vi "Sub_Seach_Changing_Point.vi"(7 "String?(F)":bool, 8 "Data Interval Time(ms)":dbl, 9 "Reverse Search?":bool, 10 "Input":string, 11 "Input Array":u32[](array[numeric])) -> (3 "Output":i32[](array[numeric]))   [LabVIEW 2015]
panel:
  out "x-y":i32[](array[numeric])
  out "Waveform Graph":u32[][](graph)
  out "Array":i32[](array[numeric])
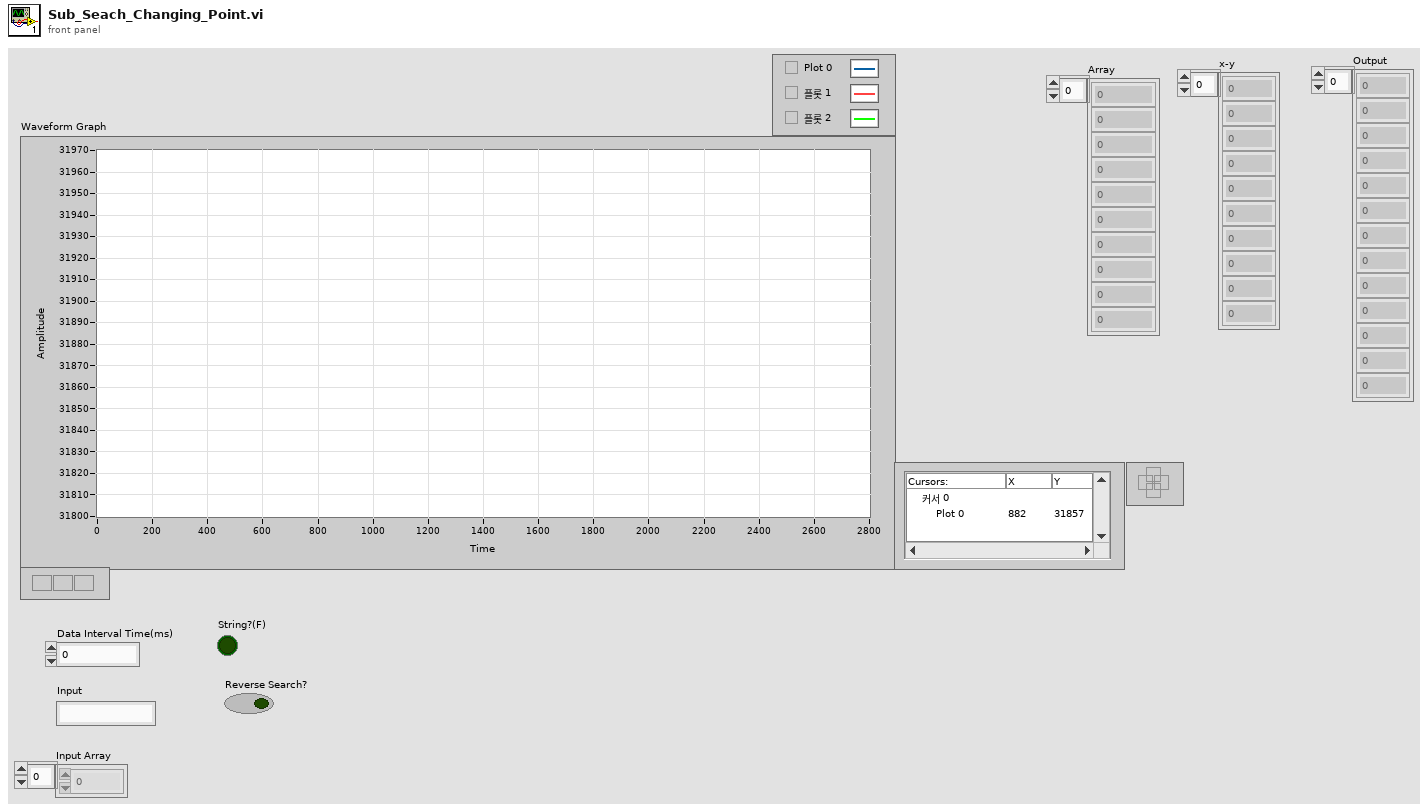
[diagram p1: front panel]
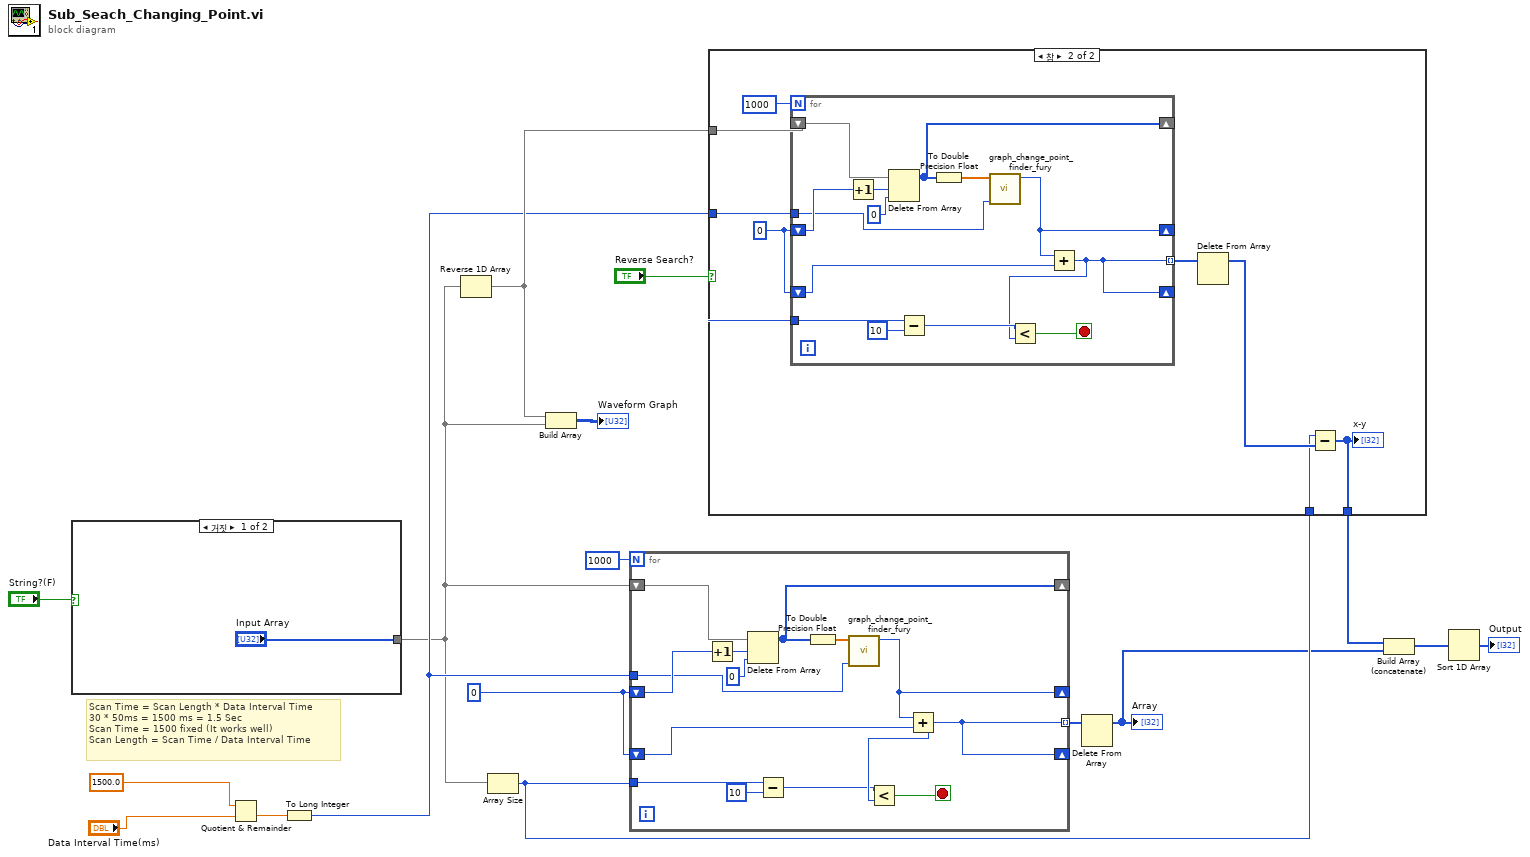
[diagram p0: block diagram]
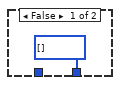
[diagram p2: hidden frame]
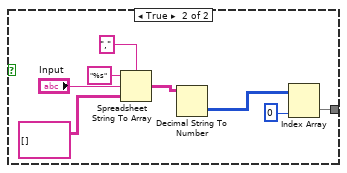
[diagram p3: hidden frame]
diagram:
  w17 = 0 ("Trace Change point")
  # "Scan Time = Scan Length * Data Interval Time\n30 * 50ms = 1500 ms = 1.5 Sec\nScan Time = 1500 fixed (It works well)\nScan Length = Scan Time / Data Interval Time"
  n1 = case shown="거짓" "String?(F)" {
    tunnel: ["Input Array" w19] -> w2
    frame False {
    }
    frame True {
      n2 = Spreadsheet String To Array(delimiter (Tab)="," ("구분 문자(탭)"), format string="%s" ("포맷 문자열"), spreadsheet string="Input", array type (2D Dbl)=string[][] []) -> (array=w22:string[][])
      n3 = Decimal String To Number(string=w22) -> (number=w20:i32[][])  [unwired: 2 in, 1 out]
      n4 = Index Array(array=w20, index (col)=0 ("disabled index (col)")) -> (element=w19:i32[])  [unwired: 1 in]
    }
  }
  n5 = Quotient & Remainder(x=1500.0, y="Data Interval Time(ms)") -> (floor(x/y)=w13:dbl)  [unwired: 1 out]
  n6 = To Long Integer(number=w13) -> (32bit integer=w10:i32)
  n7 = Reverse 1D Array(array=w2) -> (reversed array=w12:u32[])
  n8 = Array Size(array=w2) -> (size(s)=w9:i32)
  n9 = Build Array(w12, w2) -> (→"Waveform Graph":u32[][])
  n10 = for {
    N: 1000 -> [_]
    shift-right: [w34] -> _
    shift-left: w17 -> [w40]
    shift-right: [w37] -> _
    shift-left: w2 -> [w35]
    tunnel: [w33] -> w8 mode=indexing
    shift-right: [w33] -> _
    shift-left: w17 -> [w39]
    tunnel: w9 -> [w36]
    tunnel: w10 -> [w32]
    stop <- w38 stop-if-true
    n11 = Increment(x=w40) -> (x+1=w30:i32)
    n12 = Delete From Array(array=w35, length=w30, index=0 ("인덱스")) -> (array with subset deleted=w37:u32[])  [unwired: 1 out]
    n13 = Subtract(x=w36, y=10) -> (x-y=w28:i32)
    n14 = To Double Precision Float(number=w37) -> (double precision float=w27:dbl[])
    n15 = call "graph_change_point_finder_fury.vi"("Scan length"=w32, "subarray 2"=w27) -> ("Trace Change point"=w34:i32)  [unwired: 9 in]
    n16 = Add(x=w34, y=w39) -> (x+y=w33:i32)
    n17 = Less?(x=w28, y=w33) -> (x < y?=w38:bool)
  }
  n18 = case shown="참" "Reverse Search?" {
    tunnel: w12 -> [_ w46]
    tunnel: w10 -> [_ w44]
    tunnel: w9 -> [_ w43]
    tunnel: [i32[] [] w42] -> w7
    frame False {
    }
    frame True {
      w45 = 0 ("Trace Change point")
      n19 = for {
        N: 1000 -> [_]
        shift-right: [w54] -> _
        shift-left: w45 -> [w62]
        shift-right: [w58] -> _
        shift-left: w46 -> [w55]
        tunnel: [w52] -> w48 mode=indexing
        shift-right: [w52] -> _
        shift-left: w45 -> [w61]
        tunnel: w43 -> [w57]
        tunnel: w44 -> [w51]
        stop <- w59 stop-if-true
        n20 = Increment(x=w62) -> (x+1=w60:i32)
        n21 = Delete From Array(array=w55, length=w60, index=0 ("인덱스")) -> (array with subset deleted=w58:u32[])  [unwired: 1 out]
        n22 = Subtract(x=w57, y=10) -> (x-y=w53:i32)
        n23 = To Double Precision Float(number=w58) -> (double precision float=w50:dbl[])
        n24 = call "graph_change_point_finder_fury.vi"("Scan length"=w51, "subarray 2"=w50) -> ("Trace Change point"=w54:i32)  [unwired: 9 in]
        n25 = Add(x=w54, y=w61) -> (x+y=w52:i32)
        n26 = Less?(x=w53, y=w52) -> (x < y?=w59:bool)
      }
      n27 = Delete From Array(array=w48) -> (array with subset deleted=w47:i32[])  [unwired: 2 in, 1 out]
      n28 = Subtract(x=w43, y=w47) -> (x-y=w42:i32[])
      "x-y" <- w42
    }
  }
  n29 = Delete From Array(array=w8) -> (array with subset deleted=w6:i32[])  [unwired: 2 in, 1 out]
  "Array" <- w6
  n30 = Build Array (concatenate)(w7, w6) -> (w5:i32[])
  n31 = Sort 1D Array(array=w5) -> (sorted array=→"Output":i32[])
